vi "getObjectIDValue.vi"(7 "Name":string, 8 "error in (no error)":errorcluster, 11 "tBSONDocument in":refnum<class "tBSONDocument.lvclass">) -> (0 "error out":errorcluster, 2 "Value":string, 3 "tBSONDocument out":refnum<class "tBSONDocument.lvclass">)   [LabVIEW 2013, in "BSON.lvlib" / "tBSONDocument.lvclass"]
doc: "Retrieves an Object ID from a BSON document."
uses:
  tBSONDocument.lvclass
  BSONElements/tBSONObjectID/tBSONObjectID.lvclass
  BSONElements/tBSONObjectID/getValue.vi
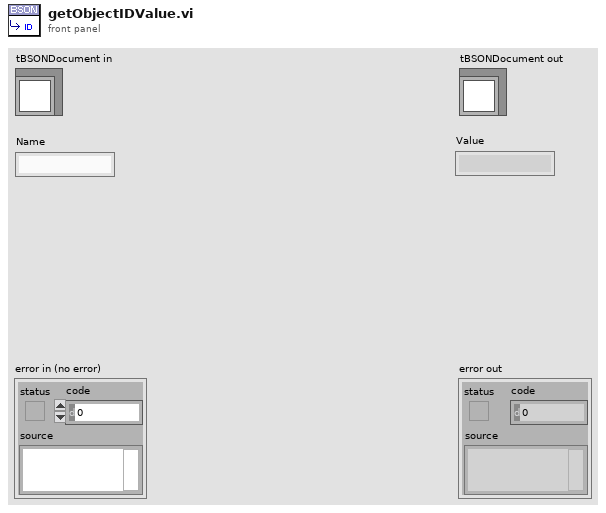
[diagram p1: front panel]
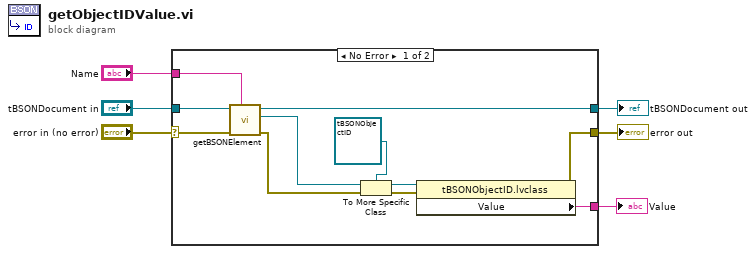
[diagram p0: block diagram]
diagram:
  n1 = case shown="No Error" "error in (no error)" {
    selector: "error in (no error)" -> [w16 w19]
    tunnel: [w10 w19] -> w3
    tunnel: [w11 w18] -> w4
    tunnel: "tBSONDocument in" -> [w17 w18]
    tunnel: "Name" -> [w8 _]
    tunnel: [w9 _] -> w2
    frame No Error {
      n2 = call "getBSONElement.vi"("Name"=w8, "error in (no error)"=w16, "tBSONDocument in"=w17) -> ("error out"=w12:errorcluster, "Element"=w13:refnum<class "tBSONElement.lvclass">, "tBSONDocument out"=w11:refnum<class "tBSONDocument.lvclass">)  [unwired: 6 in]
      n3 = To More Specific Class(target class=refnum<class "tBSONObjectID.lvclass"> refnum ("lvMongoDriver.lvlib:BSON.lvlib:tBSONObjectID.lvclass"), reference=w13, error in=w12) -> (specific class reference=w15:refnum<class "tBSONObjectID.lvclass">, error out=w14:errorcluster)
      n4 = property class="tBSONObjectID.lvclass"(reference=w15, error in=w14) -> (error out=w10:errorcluster, "Value"=w9:string)  [unwired: 1 out]
    }
    frame Error {
    }
  }
  "error out" <- w3
  "tBSONDocument out" <- w4
  "Value" <- w2
